vi "Create Spreadsheet Headers for v3.2.vi"() -> (3 "Array":string[](array[string]))   [LabVIEW 2018]
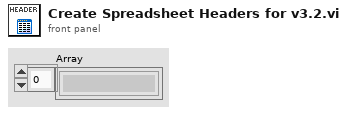
[diagram p1: front panel]
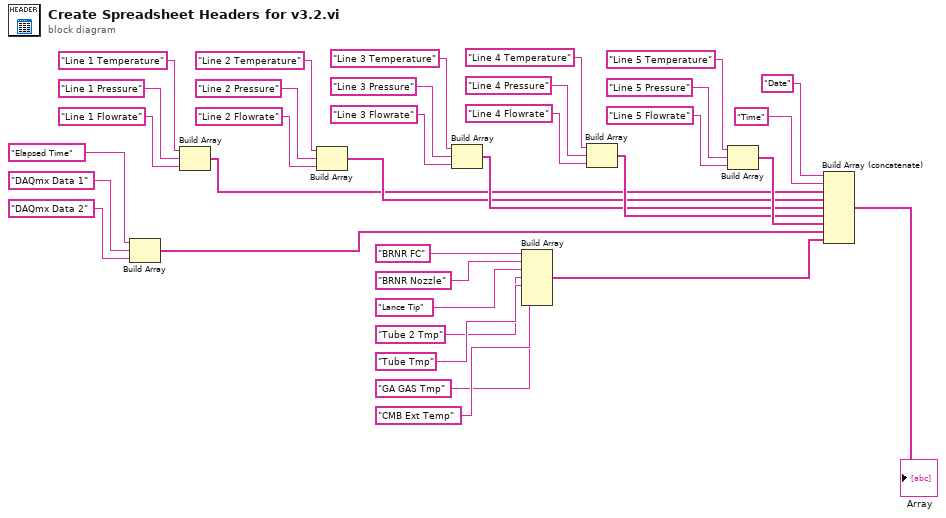
[diagram p0: block diagram]
diagram:
  n1 = Build Array("Elapsed Time", "DAQmx Data 1", "DAQmx Data 2") -> (w26:string[])
  n2 = Build Array("Line 1 Temperature", "Line 1 Pressure", "Line 1 Flowrate") -> (w17:string[])
  n3 = Build Array("Line 2 Temperature", "Line 2 Pressure", "Line 2 Flowrate") -> (w18:string[])
  n4 = Build Array("Line 3 Temperature", "Line 3 Pressure", "Line 3 Flowrate") -> (w19:string[])
  n5 = Build Array("BRNR FC", "BRNR Nozzle", "Lance Tip", "Tube 2 Tmp", "Tube Tmp", "GA GAS Tmp", "CMB Ext Temp") -> (w34:string[])
  n6 = Build Array("Line 4 Temperature", "Line 4 Pressure", "Line 4 Flowrate") -> (w20:string[])
  n7 = Build Array("Line 5 Temperature", "Line 5 Pressure", "Line 5 Flowrate") -> (w25:string[])
  n8 = Build Array (concatenate)("Date", "Time", w17, w18, w19, w20, w25, w26, w34) -> (→"Array":string[])
